vi "Get Wavelength Set Status.vi"(8 "error in":errorcluster, 11 "reference":refnum<k24>) -> (0 "error out":errorcluster, 1 "WavelengthSettingCompletionPart":dbl, 2 "IsWavelengthSettingInProgress":bool, 3 "reference out":refnum<k24>)   [LabVIEW 2020, in "Topas4.lvlib"]
uses:
  Topas4.lvlib
  C:/Windows/SysWOW64/Topas4Lib.dll
  Windows/SysWOW64/Topas4Lib.dll
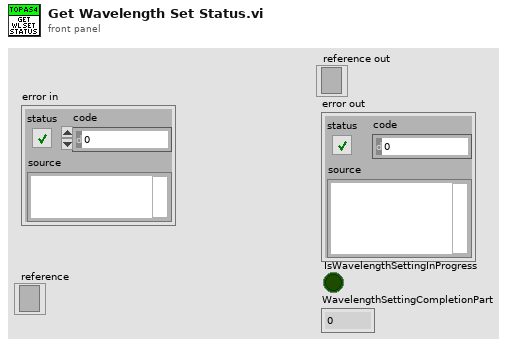
[diagram p1: front panel]
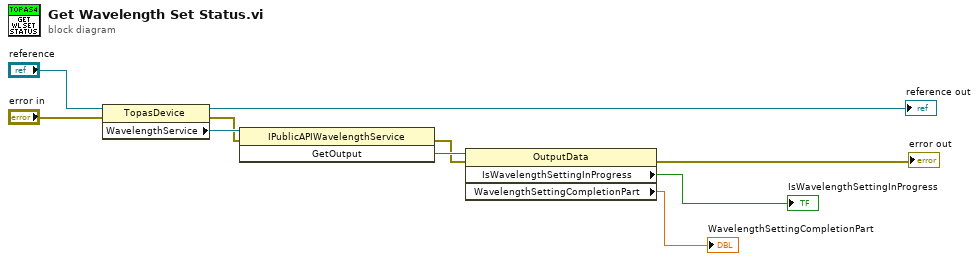
[diagram p0: block diagram]
diagram:
  n1 = property class="TopasDevice"(reference="reference", error in="error in") -> (reference out=→"reference out":refnum<k24>, error out=w6:errorcluster, "WavelengthService"=w7:refnum<k24>)
  n2 = invoke class="IPublicAPIWavelengthService" method="GetOutput"(reference=w7, error in=w6) -> (error out=w4:errorcluster, "GetOutput"=w5:refnum<k24>)  [unwired: 1 in, 1 out]
  n3 = property class="OutputData"(reference=w5, error in=w4) -> (error out=→"error out":errorcluster, "IsWavelengthSettingInProgress"=→"IsWavelengthSettingInProgress":bool, "WavelengthSettingCompletionPart"=→"WavelengthSettingCompletionPart":dbl)  [unwired: 1 out]
